vi "Fetch Multi Points.vi"(0 "VISA resource name":refnum<visa-resource-name>, 3 "Timeout (10000 ms)":i32=10000 format="%#.6g", 5 "error in (no error)":errorcluster) -> (14 "VISA resource name out":refnum<visa-resource-name>, 16 "Measurements":dbl[](array[numeric]), 19 "error out":errorcluster)   [LabVIEW 2020, in "Keithley 2100 Series.lvlib"]
doc: "This low-level VI returns an array of values from a previously initiated measurement. The number of measurements the DMM takes is determined by the values you specify for the <B>Trigger Count</B> control and <B>Sample Count</B> control of the Configure Multipoint VI.\n\n<B>Note:</B> Use this VI only with other low-level VIs. The high-level VIs automatically incorporate this functionality. This VI does not check the instrument status. If you want to check the instrument status, call the Error Query VI at the conclusion of the sequence."
uses:
  Keithley 2100 Series.lvlib
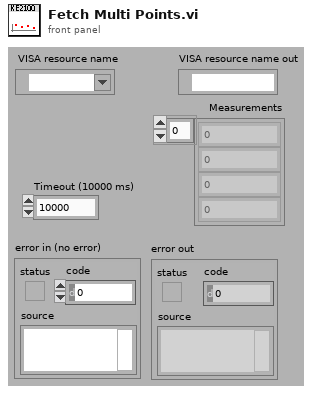
[diagram p1: front panel]
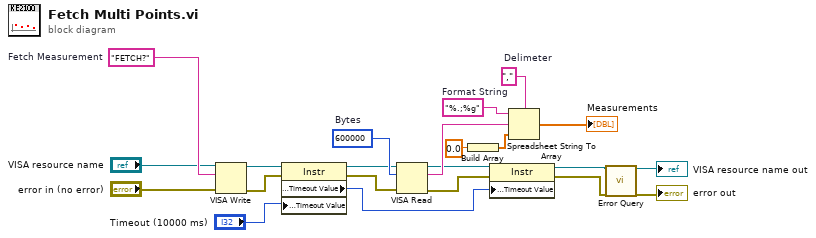
[diagram p0: block diagram]
diagram:
  w17 = ","  # Delimeter
  w18 = "%.;%g"  # Format String
  w8 = "FETCH?"  # Fetch Measurement
  w20 = u32 600000  # Bytes
  n1 = VISA Write(VISA resource name="VISA resource name", write buffer=w8, error in (no error)="error in (no error)") -> (VISA resource name out=w7:refnum<visa-resource-name>, error out=w6:errorcluster)  [unwired: 1 out]
  n2 = property class="Instr"(reference=w7, error in=w6, "General Settings:Timeout Value"="Timeout (10000 ms)") -> (reference out=w14:refnum<visa-resource-name>, error out=w13:errorcluster, "General Settings:Timeout Value"=w9:u32)
  n3 = VISA Read(VISA resource name=w14, byte count=w20, error in (no error)=w13) -> (VISA resource name out=w11:refnum<visa-resource-name>, read buffer=w19:string, error out=w10:errorcluster)  [unwired: 1 out]
  n4 = Build Array(0.0) -> (w15:dbl[])
  n5 = property class="Instr"(reference=w11, error in=w10, "General Settings:Timeout Value"=w9) -> (reference out=w5:refnum<visa-resource-name>, error out=w4:errorcluster)
  n6 = Spreadsheet String To Array(delimiter (Tab)=w17, format string=w18, spreadsheet string=w19, array type (2D Dbl)=w15) -> (array=→"Measurements":dbl[])
  n7 = call "Error Query.vi"("VISA resource name"=w5, "error in (no error)"=w4) -> ("VISA resource name out"=→"VISA resource name out":refnum<visa-resource-name>, "error out"=→"error out":errorcluster)  [unwired: 14 in, 2 out]
